vi "E816_All_VIs.vi"   [LabVIEW 2011]
doc: "This VI contains all high level and low level VIs valid for E-816. \nSee diagram for a survey of all E-816 high level and low level VIs. \nMenu / Browse / Show VI Hierarchy will show the file paths of the VIs. \nGlobal Variables are shown as Control as well as Indicator."
uses:
  Low Level/Communication.llb/Global1.vi
  Low Level/General command.llb/Controller names.ctl
  Low Level/Support.llb/Unbunde/bundle interface clusters for PI Terminal.vi
  Low Level/Communication.llb/Available DLL interfaces.ctl
  Low Level/Communication.llb/Available DLLs.ctl
  Low Level/Communication.llb/Available interfaces.ctl
  Low Level/Communication.llb/Termination character.ctl
  Low Level/General command.llb/Global2 (Array).vi
  Low Level/Communication.llb/Global DaisyChain.vi
  Low Level/Analog control.llb/Available Analog Commands.ctl
  Low Level/Analog control.llb/Global Analog.vi
  Low Level/Old commands.llb/Global2.vi
panel:
  # "E-816 PI GCS LabVIEW driver set"
  # "This VI contains all high level and low level VIs valid for E-816. See diagram for a survey\nof all E-816 high level and low level VIs. Menu / Browse / Show VI Hierarchy will show\nthe file paths of the VIs. Global Variables are shown as Control as well as Indicator."
types:
  T1 = typedef "Available Analog Commands.ctl" = enum16{"INITIALIZE", "VOL?", "VOL ", "CLOSE", "MOV", "POS?", "VCO", "VCO?", "WAIT_WF", "TMN?", "TMX?", "VEL", "VEL?", "SAI?", "MVR", "ERR?", "#24", "STP", "*IDN?", "#5", "STE", "DRR?", "W_Wave", "HLP?", "W/R_Wave"}
  T2 = typedef "Termination character.ctl" = enum16{"LF", "CR", "LFCR", "CRLF"}
  T3 = typedef "Available interfaces.ctl" = u16
  T4 = typedef "Available DLLs.ctl" = u16
  T5 = typedef "Available DLL interfaces.ctl" = u16
  T6 = typedef "Controller names.ctl" = enum16{"None", "Analog", "C-702", "C-843", "C-843.PM", "C-844", "C-848", "C-865", "C-866", "C-880", "E-516", "E-710", "E-712", "E-725", "E-753", "E-755", "E-761", "E-816", "F-206", "M-840", "M-850", "M-8X0", "Mercury"}
  T7 = cluster{"Conversion factor":dbl[], "Velocity":dbl[], "Velocity control mode":bool, "AO.Resolution":dbl, "Lower voltage limit (V)":dbl, "Upper voltage limit (V)":dbl, "AO_WF_T (s)":dbl, "AI Sample Rate":dbl, "AI Samples/Channel":i32, "Hyperbit":bool, "Offset (V)":dbl[], "Hyperbit StayOnPos":bool, "Gain (V)":dbl[], "Bit rate (Hz)":dbl, "PWM rate (Hz)":dbl, "HyperBit Password":string, "AO.MaxRate":dbl}[]
  T8 = cluster{"No. of devices":i32, "Port ID":i32, "Devices":string[], "Description":string}[]
  T9 = cluster{"Conn. axes":string[], "Controller name":T6}[]
  T10 = cluster{"System 1":string[], "System 2":string[], "System 3":string[], "System 4":string[]}
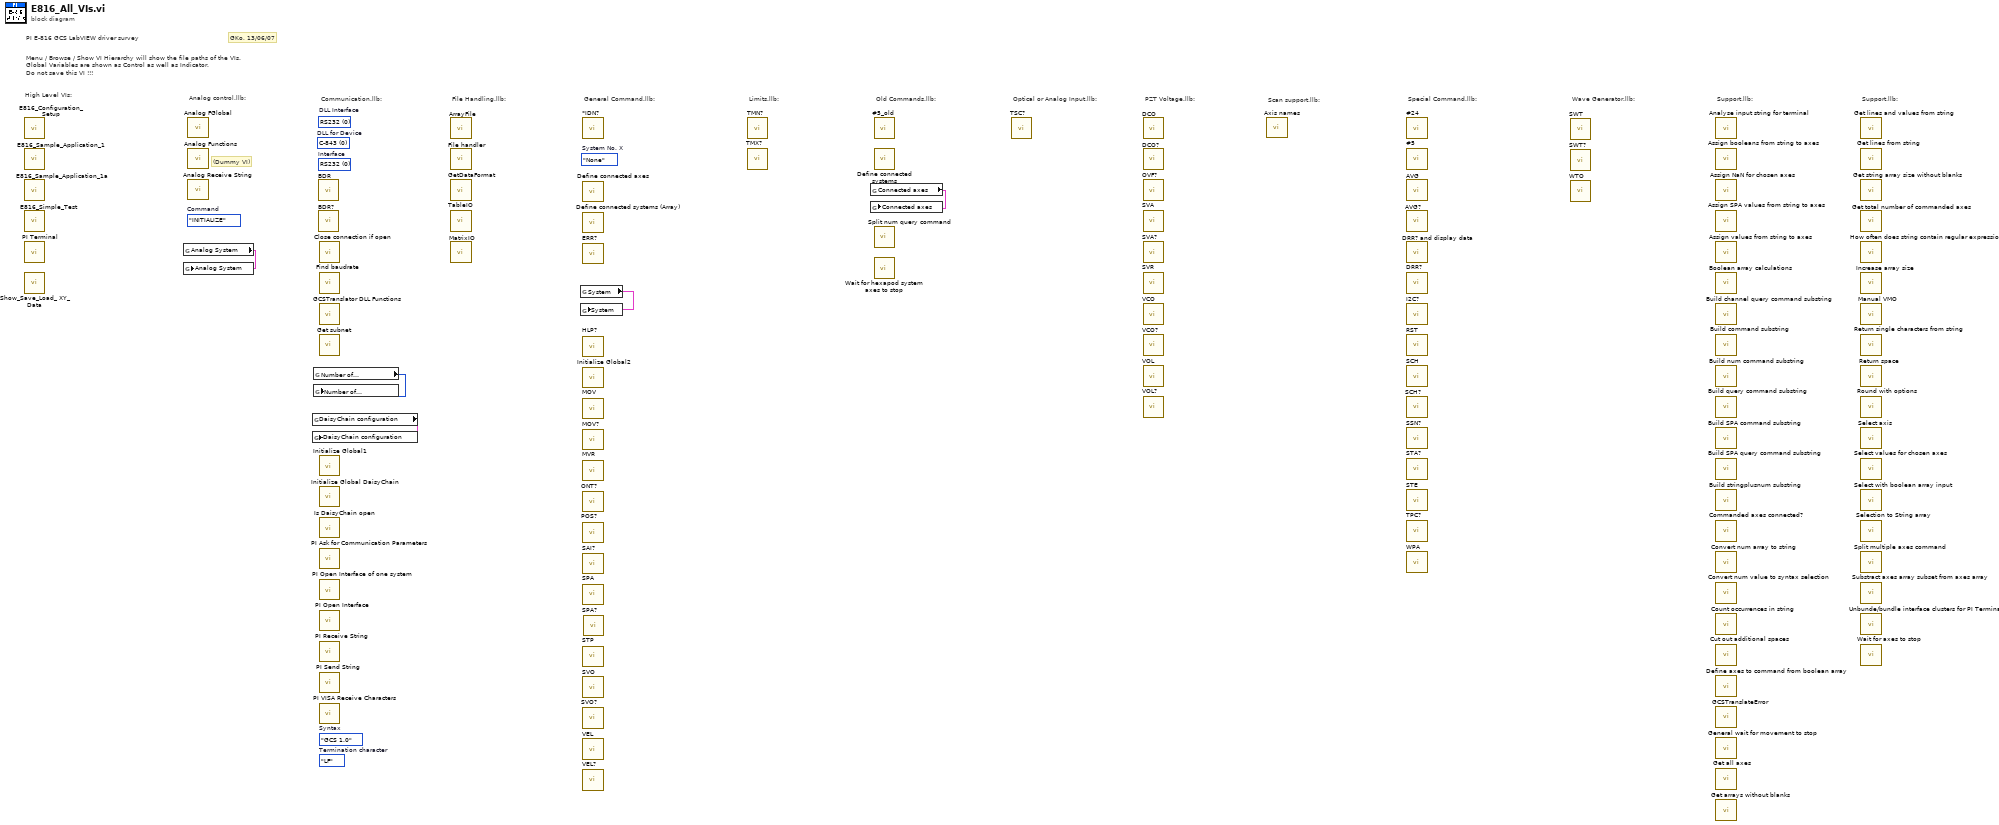
[diagram p0: block diagram]
diagram:
  (unwired) Available_Analog_Commands."INITIALIZE"  # Command
  (unwired) Termination_character."LF"  # Termination character
  (unwired) enum16{"GCS 1.0", "GCS 2.0"}."GCS 1.0"  # Syntax
  (unwired) T3 0 items=["RS232", "GPIB", "DLL", "TCP-IP"]  # Interface
  (unwired) T4 0 items=["C-843", "C-844", "E-710", "C-843.PM", "C-865", "E-761", "Mercury"]  # DLL for Device
  (unwired) T5 0 items=["RS232", "GPIB", "Board", "TCP-IP", "USB"]  # DLL Interface
  (unwired) Controller_names."None"  # System No. X
  # "Scan support.llb:"
  # "(Dummy VI)"
  # "GKo, 13/06/07"
  # "High Level VIs:"
  # "Analog control.llb:"
  # "Support.llb:"
  # "Wave Generator.llb:"
  # "Support.llb:"
  # "Special Command.llb:"
  # "PZT Voltage.llb:"
  # "Optical or Analog Input.llb:"
  # "Old Commands.llb:"
  # "Limits.llb:"
  # "General Command.llb:"
  # "File Handling.llb:"
  # "Menu / Browse / Show VI Hierarchy will show the file paths of the VIs. \nGlobal Variables are shown as Control as well as Indicator.\nDo not save this VI !!!"
  # "PI E-816 GCS LabVIEW driver survey"
  # "Communication.llb:"
  n1 = call "E816_Configuration_Setup.vi"() -> ()  [unwired: 16 in, 4 out]
  n2 = call "E816_Sample_Application_1.vi"() -> ()  [unwired: 20 in]
  n3 = call "E816_Sample_Application_1a.vi"() -> ()  [unwired: 20 in]
  n4 = call "E816_Simple_Test.vi"() -> ()  [unwired: 20 in]
  n5 = call "PI Terminal.vi"() -> ()  [unwired: 20 in]
  n6 = call "Show_Save_Load_ XY_Data.vi"() -> ()  [unwired: 19 in, 1 out]
  n7 = global read "Global Analog.vi" "Analog System"() -> (w2:T7)
  n8 = global write "Global Analog.vi" "Analog System"(w2) -> ()
  n9 = call "Analog FGlobal.vi"() -> ()  [unwired: 19 in, 1 out]
  n10 = call "Analog Functions.vi"() -> ()  [unwired: 17 in, 3 out]
  n11 = call "Analog Receive String.vi"() -> ()  [unwired: 18 in, 2 out]
  n12 = global read "Global DaisyChain.vi" "DaisyChain configuration"() -> (w3:T8)
  n13 = global write "Global DaisyChain.vi" "DaisyChain configuration"(w3) -> ()
  n14 = global read "Global1.vi" "Number of\nsystems"() -> (w5:i32)
  n15 = global write "Global1.vi" "Number of\nsystems"(w5) -> ()
  n16 = call "BDR.vi"() -> ()  [unwired: 19 in, 1 out]
  n17 = call "BDR?.vi"() -> ()  [unwired: 18 in, 2 out]
  n18 = call "Close connection if open.vi"() -> ()  [unwired: 18 in, 2 out]
  n19 = call "Find baudrate.vi"() -> ()  [unwired: 17 in, 3 out]
  n20 = call "GCSTranslator DLL Functions.vi"() -> ()  [unwired: 15 in, 5 out]
  n21 = call "Get subnet.vi"() -> ()  [unwired: 19 in, 1 out]
  n22 = call "Initialize Global1.vi"() -> ()  [unwired: 19 in, 1 out]
  n23 = call "Initialize Global DaisyChain.vi"() -> ()  [unwired: 19 in, 1 out]
  n24 = call "Is DaisyChain open.vi"() -> ()  [unwired: 17 in, 3 out]
  n25 = call "PI Ask for Communication Parameters.vi"() -> ()  [unwired: 12 in, 8 out]
  n26 = call "PI Open Interface of one system.vi"() -> ()  [unwired: 18 in, 2 out]
  n27 = call "PI Open Interface.vi"() -> ()  [unwired: 18 in, 2 out]
  n28 = call "PI Receive String.vi"() -> ()  [unwired: 17 in, 3 out]
  n29 = call "PI Send String.vi"() -> ()  [unwired: 19 in, 1 out]
  n30 = call "PI VISA Receive Characters.vi"() -> ()  [unwired: 17 in, 3 out]
  n31 = call "ArrayFile.vi"() -> ()  [unwired: 18 in, 2 out]
  n32 = call "File handler.vi"() -> ()  [unwired: 17 in, 3 out]
  n33 = call "GetDataFormat.vi"() -> ()  [unwired: 12 in, 8 out]
  n34 = call "TableIO.vi"() -> ()  [unwired: 14 in, 6 out]
  n35 = call "MatrixIO.vi"() -> ()  [unwired: 13 in, 7 out]
  n36 = global read "Global2 (Array).vi" "System"() -> (w4:T9)
  n37 = global write "Global2 (Array).vi" "System"(w4) -> ()
  n38 = call "*IDN?.vi"() -> ()  [unwired: 18 in, 2 out]
  n39 = call "Define connected axes.vi"() -> ()  [unwired: 18 in, 2 out]
  n40 = call "Define connected systems (Array).vi"() -> ()  [unwired: 19 in, 1 out]
  n41 = call "ERR?.vi"() -> ()  [unwired: 18 in, 2 out]
  n42 = call "HLP?.vi"() -> ()  [unwired: 18 in, 2 out]
  n43 = call "Initialize Global2.vi"() -> ()  [unwired: 19 in, 1 out]
  n44 = call "MOV.vi"() -> ()  [unwired: 19 in, 1 out]
  n45 = call "MOV?.vi"() -> ()  [unwired: 18 in, 2 out]
  n46 = call "MVR.vi"() -> ()  [unwired: 19 in, 1 out]
  n47 = call "ONT?.vi"() -> ()  [unwired: 18 in, 2 out]
  n48 = call "POS?.vi"() -> ()  [unwired: 18 in, 2 out]
  n49 = call "SAI?.vi"() -> ()  [unwired: 18 in, 2 out]
  n50 = call "SPA.vi"() -> ()  [unwired: 18 in, 2 out]
  n51 = call "STP.vi"() -> ()  [unwired: 19 in, 1 out]
  n52 = call "SVO.vi"() -> ()  [unwired: 19 in, 1 out]
  n53 = call "SVO?.vi"() -> ()  [unwired: 18 in, 2 out]
  n54 = call "VEL.vi"() -> ()  [unwired: 18 in, 2 out]
  n55 = call "VEL?.vi"() -> ()  [unwired: 18 in, 2 out]
  n56 = call "SPA?.vi"() -> ()  [unwired: 17 in, 3 out]
  n57 = call "TMN?.vi"() -> ()  [unwired: 18 in, 2 out]
  n58 = call "TMX?.vi"() -> ()  [unwired: 18 in, 2 out]
  n59 = global read "Global2.vi" "Connected axes"() -> (w1:T10)
  n60 = global write "Global2.vi" "Connected axes"(w1) -> ()
  n61 = call "#5_old.vi"() -> ()  [unwired: 16 in, 4 out]
  n62 = call "Define connected systems.vi"() -> ()  [unwired: 18 in, 2 out]
  n63 = call "Split num query command.vi"() -> ()  [unwired: 18 in, 2 out]
  n64 = call "Wait for hexapod system axes to stop.vi"() -> ()  [unwired: 18 in, 2 out]
  n65 = call "TSC?.vi"() -> ()  [unwired: 18 in, 2 out]
  n66 = call "DCO.vi"() -> ()  [unwired: 19 in, 1 out]
  n67 = call "DCO?.vi"() -> ()  [unwired: 18 in, 2 out]
  n68 = call "OVF?.vi"() -> ()  [unwired: 18 in, 2 out]
  n69 = call "SVA.vi"() -> ()  [unwired: 19 in, 1 out]
  n70 = call "SVA?.vi"() -> ()  [unwired: 18 in, 2 out]
  n71 = call "SVR.vi"() -> ()  [unwired: 19 in, 1 out]
  n72 = call "VCO.vi"() -> ()  [unwired: 19 in, 1 out]
  n73 = call "VCO?.vi"() -> ()  [unwired: 18 in, 2 out]
  n74 = call "VOL.vi"() -> ()  [unwired: 19 in, 1 out]
  n75 = call "VOL?.vi"() -> ()  [unwired: 18 in, 2 out]
  n76 = call "Axis names.vi"() -> ()  [unwired: 17 in, 3 out]
  n77 = call "#24.vi"() -> ()  [unwired: 19 in, 1 out]
  n78 = call "#5.vi"() -> ()  [unwired: 18 in, 2 out]
  n79 = call "AVG.vi"() -> ()  [unwired: 18 in, 2 out]
  n80 = call "AVG?.vi"() -> ()  [unwired: 18 in, 2 out]
  n81 = call "DRR? and display data.vi"() -> ()  [unwired: 16 in, 4 out]
  n82 = call "DRR?.vi"() -> ()  [unwired: 16 in, 4 out]
  n83 = call "I2C?.vi"() -> ()  [unwired: 18 in, 2 out]
  n84 = call "RST.vi"() -> ()  [unwired: 19 in, 1 out]
  n85 = call "SCH.vi"() -> ()  [unwired: 19 in, 1 out]
  n86 = call "SCH?.vi"() -> ()  [unwired: 18 in, 2 out]
  n87 = call "SSN?.vi"() -> ()  [unwired: 18 in, 2 out]
  n88 = call "STA?.vi"() -> ()  [unwired: 18 in, 2 out]
  n89 = call "STE.vi"() -> ()  [unwired: 19 in, 1 out]
  n90 = call "TPC?.vi"() -> ()  [unwired: 18 in, 2 out]
  n91 = call "WPA.vi"() -> ()  [unwired: 18 in, 2 out]
  n92 = call "SWT.vi"() -> ()  [unwired: 18 in, 2 out]
  n93 = call "SWT?.vi"() -> ()  [unwired: 18 in, 2 out]
  n94 = call "WTO.vi"() -> ()  [unwired: 19 in, 1 out]
  n95 = call "Analyse input string for terminal.vi"() -> ()  [unwired: 17 in, 3 out]
  n96 = call "Assign booleans from string to axes.vi"() -> ()  [unwired: 18 in, 2 out]
  n97 = call "Assign NaN for chosen axes.vi"() -> ()  [unwired: 19 in, 1 out]
  n98 = call "Assign SPA values from string to axes.vi"() -> ()  [unwired: 14 in, 6 out]
  n99 = call "Assign values from string to axes.vi"() -> ()  [unwired: 16 in, 4 out]
  n100 = call "Boolean array calculations.vi"() -> ()  [unwired: 19 in, 1 out]
  n101 = call "Build channel query command substring.vi"() -> ()  [unwired: 16 in, 4 out]
  n102 = call "Build command substring.vi"() -> ()  [unwired: 19 in, 1 out]
  n103 = call "Build num command substring.vi"() -> ()  [unwired: 19 in, 1 out]
  n104 = call "Build query command substring.vi"() -> ()  [unwired: 17 in, 3 out]
  n105 = call "Build SPA command substring.vi"() -> ()  [unwired: 19 in, 1 out]
  n106 = call "Build SPA query command substring.vi"() -> ()  [unwired: 18 in, 2 out]
  n107 = call "Build stringplusnum substring.vi"() -> ()  [unwired: 18 in, 2 out]
  n108 = call "Commanded axes connected?.vi"() -> ()  [unwired: 18 in, 2 out]
  n109 = call "Convert num array to string.vi"() -> ()  [unwired: 19 in, 1 out]
  n110 = call "Convert num value to syntax selection.vi"() -> ()  [unwired: 19 in, 1 out]
  n111 = call "Count occurrences in string.vi"() -> ()  [unwired: 19 in, 1 out]
  n112 = call "Cut out additional spaces.vi"() -> ()  [unwired: 19 in, 1 out]
  n113 = call "Define axes to command from boolean array.vi"() -> ()  [unwired: 17 in, 3 out]
  n114 = call "GCSTranslateError.vi"() -> ()  [unwired: 17 in, 3 out]
  n115 = call "General wait for movement to stop.vi"() -> ()  [unwired: 18 in, 2 out]
  n116 = call "Get all axes.vi"() -> ()  [unwired: 19 in, 1 out]
  n117 = call "Get arrays without blanks.vi"() -> ()  [unwired: 16 in, 4 out]
  n118 = call "Get lines and values from string.vi"() -> ()  [unwired: 17 in, 3 out]
  n119 = call "Get lines from string.vi"() -> ()  [unwired: 18 in, 2 out]
  n120 = call "Get string array size without blanks.vi"() -> ()  [unwired: 19 in, 1 out]
  n121 = call "Get total number of commanded axes.vi"() -> ()  [unwired: 16 in, 4 out]
  n122 = call "How often does string contain regular expression?.vi"() -> ()  [unwired: 19 in, 1 out]
  n123 = call "Increase array size.vi"() -> ()  [unwired: 19 in, 1 out]
  n124 = call "Manual VMO.vi"() -> ()  [unwired: 18 in, 2 out]
  n125 = call "Return single characters from string.vi"() -> ()  [unwired: 18 in, 2 out]
  n126 = call "Return space.vi"() -> ()  [unwired: 18 in, 2 out]
  n127 = call "Round with options.vi"() -> ()  [unwired: 18 in, 2 out]
  n128 = call "Select axis.vi"() -> ()  [unwired: 18 in, 2 out]
  n129 = call "Select values for chosen axes.vi"() -> ()  [unwired: 19 in, 1 out]
  n130 = call "Select with boolean array input.vi"() -> ()  [unwired: 19 in, 1 out]
  n131 = call "Selection to String array.vi"() -> ()  [unwired: 19 in, 1 out]
  n132 = call "Split multiple axes command.vi"() -> ()  [unwired: 17 in, 3 out]
  n133 = call "Substract axes array subset from axes array.vi"() -> ()  [unwired: 18 in, 2 out]
  n134 = call "Unbunde/bundle interface clusters for PI Terminal.vi"() -> ()  [unwired: 13 in, 7 out]
  n135 = call "Wait for axes to stop.vi"() -> ()  [unwired: 18 in, 2 out]
